vi "Stop Core.vi"(10 "final error code":i32, 11 "Instruments in":refnum<class "Instruments.lvclass">) -> (3 "Instruments out":refnum<class "Instruments.lvclass">)   [LabVIEW 2023, in "Instruments.lvlib" / "Instruments.lvclass"]
uses:
  Library/Instruments.lvclass
  builds/Tools/Config.lvlibp/Config.lvclass
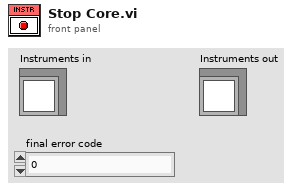
[diagram p1: front panel]
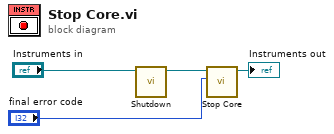
[diagram p0: block diagram]
diagram:
  n1 = call-dynamic "Shutdown.vi"("Instruments in"="Instruments in") -> ("Instruments out"=w1:refnum<class "Instruments.lvclass">)  [unwired: 9 in, 1 out]
  n2 = call-parent "Stop Core.vi"("final error code"="final error code", "Monitored Actor in"=w1) -> ("Monitored Actor out"=→"Instruments out":refnum<class "Instruments.lvclass">)  [unwired: 9 in]
